vi "Get Display Text.vi"(8 "error in (no error)":errorcluster, 11 "Attribute in":refnum<class "Attribute.lvclass">) -> (0 "error out":errorcluster, 1 "Detail Text":string, 2 "Display Name":string, 3 "Attribute out":refnum<class "Attribute.lvclass">)   [LabVIEW 2026, in "VILab.lvlib" / "Attribute.lvclass"]
uses:
  Attribute.lvclass
  Attribute.lvclass/Attribute.ctl
  Data Item/Data Item.lvclass
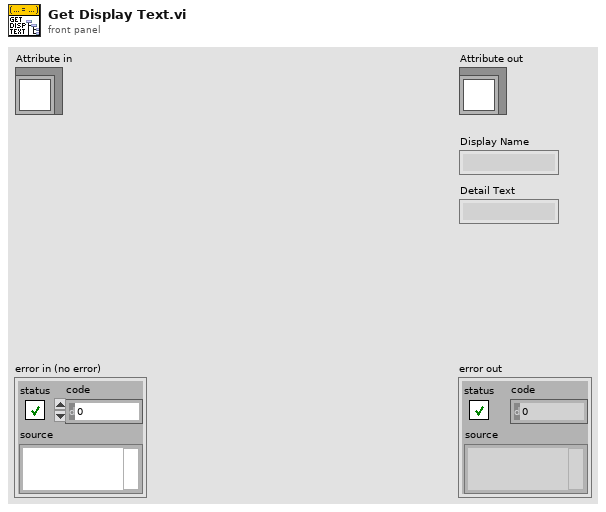
[diagram p1: front panel]
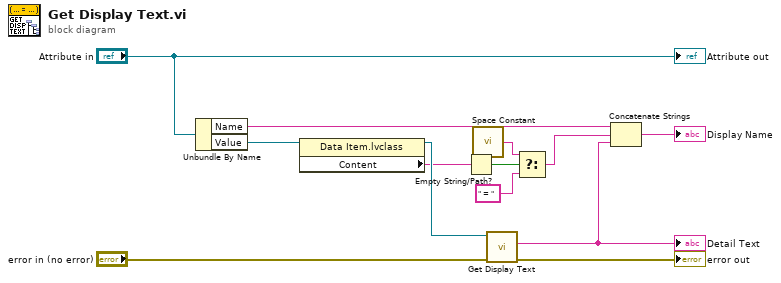
[diagram p0: block diagram]
diagram:
  n1 = Unbundle By Name("Attribute in") -> ("Name"=w10:string, "Value"=w7:refnum<class "Data Item.lvclass">)
  n2 = property class="Data Item.lvclass"(reference=w7) -> (reference out=w6:refnum<class "Data Item.lvclass">, "Content"=w5:string)  [unwired: 1 in, 1 out]
  n3 = Empty String/Path?(string/path=w5) -> (empty?=w4:bool)
  n4 = call <vilib>:"Space Constant.vi"() -> ("String"=w3:string)
  n5 = call-dynamic "Get Display Text.vi"("error in (no error)"="error in (no error)", "Data Item in"=w6) -> ("error out"=→"error out":errorcluster, "Display Name"=w9:string)  [unwired: 6 in, 2 out]
  "Detail Text" <- w9
  n6 = Select(t=w3, s=w4, f=" = ") -> (s? t:f=w1:string)
  n7 = Concatenate Strings(w10, w1, w9) -> (→"Display Name":string)
  "Attribute out" <- "Attribute in"
